vi "PH_BlackBox.ProcEvents.vi"(0 "i ref in":refnum<vi>, 5 "error in (no error)":errorcluster) -> (14 "i ref out":refnum<vi>, 19 "error out":errorcluster)   [LabVIEW 2014, in "PH_BlackBox.lvlib"]
doc: "This method is used to define the events the object will listen to. Add your own events here."
uses:
  PH_BlackBox.lvlib
  CS_Core/BaseProcess/BaseProcess.event definition.ctl
  CS_Core/CAEObj/CAEObj.event definition.ctl
  CS_Core/BaseProcess/BaseProcess.descriptor string definition.ctl
  CS_Core/BaseProcess/BaseProcess.lvlib
  CS_Core/CAEObj/CAEObj.lvlib
  PH_Basics/PH_Common/PH_Common.lvlib
  PH_Devices/PH_Beckhoff_Common/PH_Beckhoff_Common.lvlib
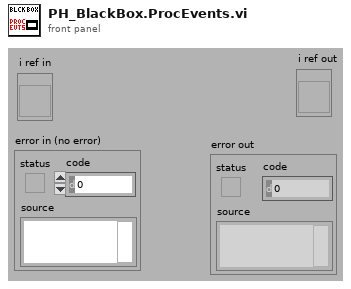
[diagram p1: front panel]
types:
  T1 = typedef "BaseProcess.lvlib/BaseProcess.event definition.ctl" = cluster{"CAEEvtDef":T2, "Data Descriptor":T3}
  T2 = typedef "CAEObj.lvlib/CAEObj.event definition.ctl" = cluster{"URL":string, "enable":bool, "ignoreResID":bool}
  T3 = typedef "BaseProcess.lvlib/BaseProcess.descriptor string definition.ctl" = string
  T4 = typedef "PH_BlackBox.lvlib/PH_BlackBox.i attribute.ctl" = cluster{"BB Remote Controlled?":bool, "GUI Refs":T5, "Position IN":T6, "Position OUT":T6, "BB Remote Controlled by other Instance?":bool, "Recipient":string, "Number":i32, "Caption Move":string, "Caption Out":string, "Caption In":string}
  T5 = typedef "PH_BlackBox.lvlib/PH_BlackBox.GUI Refs.ctl" = cluster{"MOVE IN":refnum<vi>, "MOVE":refnum<vi>, "IN":refnum<vi>, "OUT":refnum<vi>, "REMOTE":refnum<vi>, "GUI-Knob Move":refnum<vi>, "GUI-Knob Move in":refnum<vi>, "POWER ON":refnum<vi>, "Delete":refnum<vi>, "Function Textfield":refnum<vi>}
  T6 = typedef "PH_StatusHandler.lvlib/PH_StatusHandler.Status.ctl" = i16
  T7 = typedef "PH_Beckhoff_Common.lvlib/PH_Beckhoff_Common.BB Tagnames.ctl" = cluster{"Sensor Remote controlled":string, "Sensor Out":string, "Sensor In":string, "Actor Direction In":string, "Actor Move":string, "Sensor Power ok":string, "Instance":string}
  T8 = typedef "PH_Common.lvlib/PH_DIM.Event Declarer.ctl" = cluster{"Service Name":string, "Selector":string}
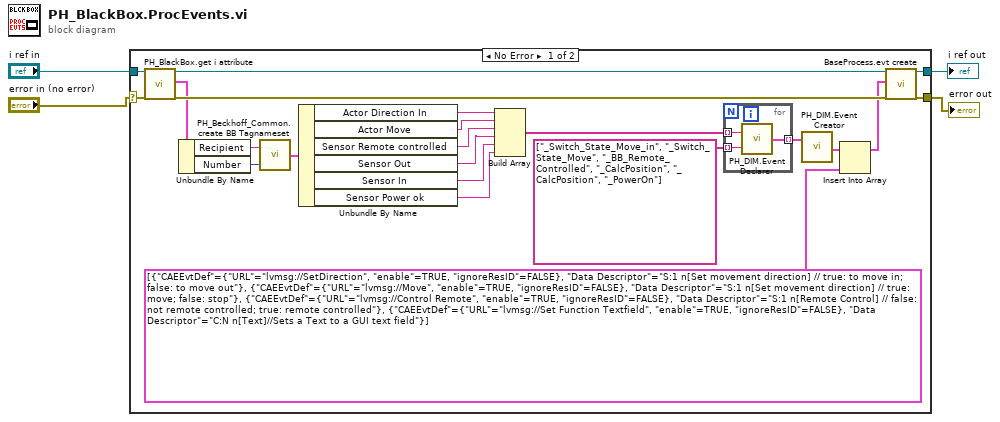
[diagram p0: block diagram]
diagram:
  n1 = case shown="No Error" "error in (no error)" {
    selector: "error in (no error)" -> [w16 w30]
    tunnel: "i ref in" -> [w26 w31]
    tunnel: [w23 w30] -> w3
    tunnel: [w22 w31] -> w2
    frame No Error {
      n2 = call "PH_BlackBox.get i attribute.vi"("i ref in"=w26, "error in (no error)"=w16) -> ("i ref out"=w24:refnum<vi>, "i attribute"=w7:T4, "error out"=w25:errorcluster)  [unwired: 15 in]
      n3 = Unbundle By Name(w7) -> ("Recipient"=w6:string, "Number"=w5:i32)
      n4 = call "PH_Beckhoff_Common.create BB Tagnameset.vi"("#"=w5, "Instance Name"=w6) -> ("output cluster"=w14:T7)
      n5 = Unbundle By Name(w14) -> ("Actor Direction In"=w8:string, "Actor Move"=w9:string, "Sensor Remote controlled"=w10:string, "Sensor Out"=w11:string, "Sensor In"=w12:string, "Sensor Power ok"=w13:string)
      n6 = Build Array(w8, w9, w10, w11, w12, w13) -> (w20:string[])
      n7 = for {
        tunnel: [w29] -> w21 mode=indexing
        tunnel: w20 -> [w28] mode=indexing
        tunnel: string[] ["_Switch_State_Move_in", "_Switch_State_Move", "_BB_Remote_Controlled", "_CalcPosition", "_CalcPosition", "_PowerOn"] -> [w27] mode=indexing
        n8 = call "PH_DIM.Event Declarer.vi"("Selector"=w27, "Service Name"=w28) -> ("declared DIM Event"=w29:T8)
      }
      n9 = call "PH_DIM.Event Creator.vi"("Trendmessage Services"=w21) -> ("DIM Service Events"=w18:T1[])  [unwired: 18 in]
      n10 = Insert Into Array(array=w18, new element=T1[] [{"CAEEvtDef"={"URL"="lvmsg://SetDirection", "enable"=TRUE, "ignoreResID"=FALSE}, "Data Descriptor"="S:1 n[Set movement direction] // true: to move in; false: to move out"}, {"CAEEvtDef"={"URL"="lvmsg://Move", "enable"=TRUE, "ignoreResID"=FALSE}, "Data Descriptor"="S:1 n[Set movement direction] // true: move; false: stop"}, {"CAEEvtDef"={"URL"="lvmsg://Control Remote", "enable"=TRUE, "ignoreResID"=FALSE}, "Data Descriptor"="S:1 n[Remote Control] // false: not remote controlled; true: remote controlled"}, {"CAEEvtDef"={"URL"="lvmsg://Set Function Textfield", "enable"=TRUE, "ignoreResID"=FALSE}, "Data Descriptor"="C:N n[Text]//Sets a Text to a GUI text field"}] ("new events")) -> (w17:T1[])  [unwired: 1 in]
      n11 = call "BaseProcess.evt create.vi"("i ref in"=w24, "newEvents"=w17, "error in (no error)"=w25) -> ("i ref out"=w22:refnum<vi>, "error out"=w23:errorcluster)  [unwired: 13 in, 2 out]
    }
    frame Error {
    }
  }
  "i ref out" <- w2
  "error out" <- w3
